vi "DrawTopMenuItems.vi"(7 "Collection in":refnum<class "Collection.lvclass">, 8 "error in (no error)":errorcluster, 10 "Coords":T2, 11 "Menu in":refnum<class "Menu.lvclass">) -> (0 "error out":errorcluster, 1 "SubMenu":bool, 2 "Area out":T1, 3 "Menu out":refnum<class "Menu.lvclass">, 4 "SelectedItemTeg":string, 5 "Collection out":refnum<class "Collection.lvclass">)   [LabVIEW 2021, in "Menu.lvlib" / "Menu.lvclass"]
uses:
  Menu.lvclass
  Menu.lvclass/Menu.ctl
  Picture2D/src/Text/Text.lvclass
  Picture2D/src/PointSpecialized/PointSpecialized.lvclass
  Picture2D/src/Rectangle/Rectangle.lvclass
  Picture2D/src/Collection/Collection.lvclass
  C:/GitHub/Picture2D/src/Point/Point.lvclass
  C:/GitHub/Picture2D/src/IDrawable/IDrawable.lvclass
  C:/GitHub/Picture2D/src/IMovable/IMovable.lvclass
  C:/GitHub/Picture2D/src/IRotatable/IRotatable.lvclass
  C:/GitHub/Picture2D/src/IScalable/IScalable.lvclass
  C:/GitHub/Picture2D/src/PointSpecialized/PointSpecialized.lvclass
  C:/GitHub/Picture2D/src/Polygone/Polygone.lvclass
  C:/GitHub/Picture2D/src/Shape/Shape.lvclass
  C:/GitHub/Picture2D/src/Picture2D/Picture2D.lvclass
  C:/GitHub/Picture2D/src/Rectangle/Rectangle.lvclass
  C:/GitHub/Picture2D/src/Text/Text.lvclass
  <vilib>/Utility/miscctls.llb/LVPoint32TypeDef.ctl
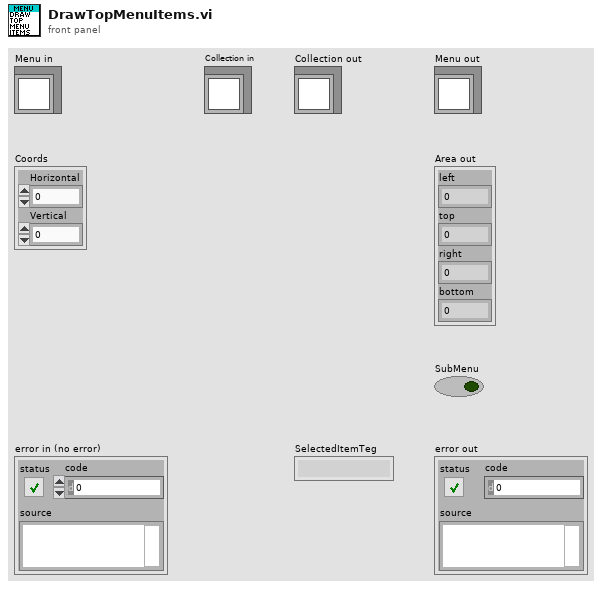
[diagram p1: front panel]
types:
  T1 = cluster{"left":i16, "top":i16, "right":i16, "bottom":i16}
  T2 = typedef "LVPoint32TypeDef.ctl" = cluster{"Horizontal":i32, "Vertical":i32}
  T3 = typedef "Menu.lvlib/Menu.lvclass/MenuItems.ctl" = cluster{"Item Name":string, "Short Cut":T4, "Checked":bool, "Enable":bool, "After item":string, "Item Tags":string[], "Item Names":string[], "Picture":refnum<class "Image.lvclass">, "Hilite Picture":refnum<class "Image.lvclass">, "Displayed":bool}
  T4 = typedef "LVMenuShortCut.ctl" = cluster{"Include Shift Key?":bool, "Include Ctrl Key?":bool, "Shortcut Key":string}
  T5 = typedef "Menu.lvlib/Menu.lvclass/MenuColors.ctl" = cluster{"Text":refnum<class "Color.lvclass">, "HiliteText":refnum<class "Color.lvclass">, "Background":refnum<class "Color.lvclass">, "BorderColor":refnum<class "Color.lvclass">, "Hilite":refnum<class "Color.lvclass">}
  T6 = enum16{"User-specified Font", "Application Font", "System Font", "Dialog Font"}
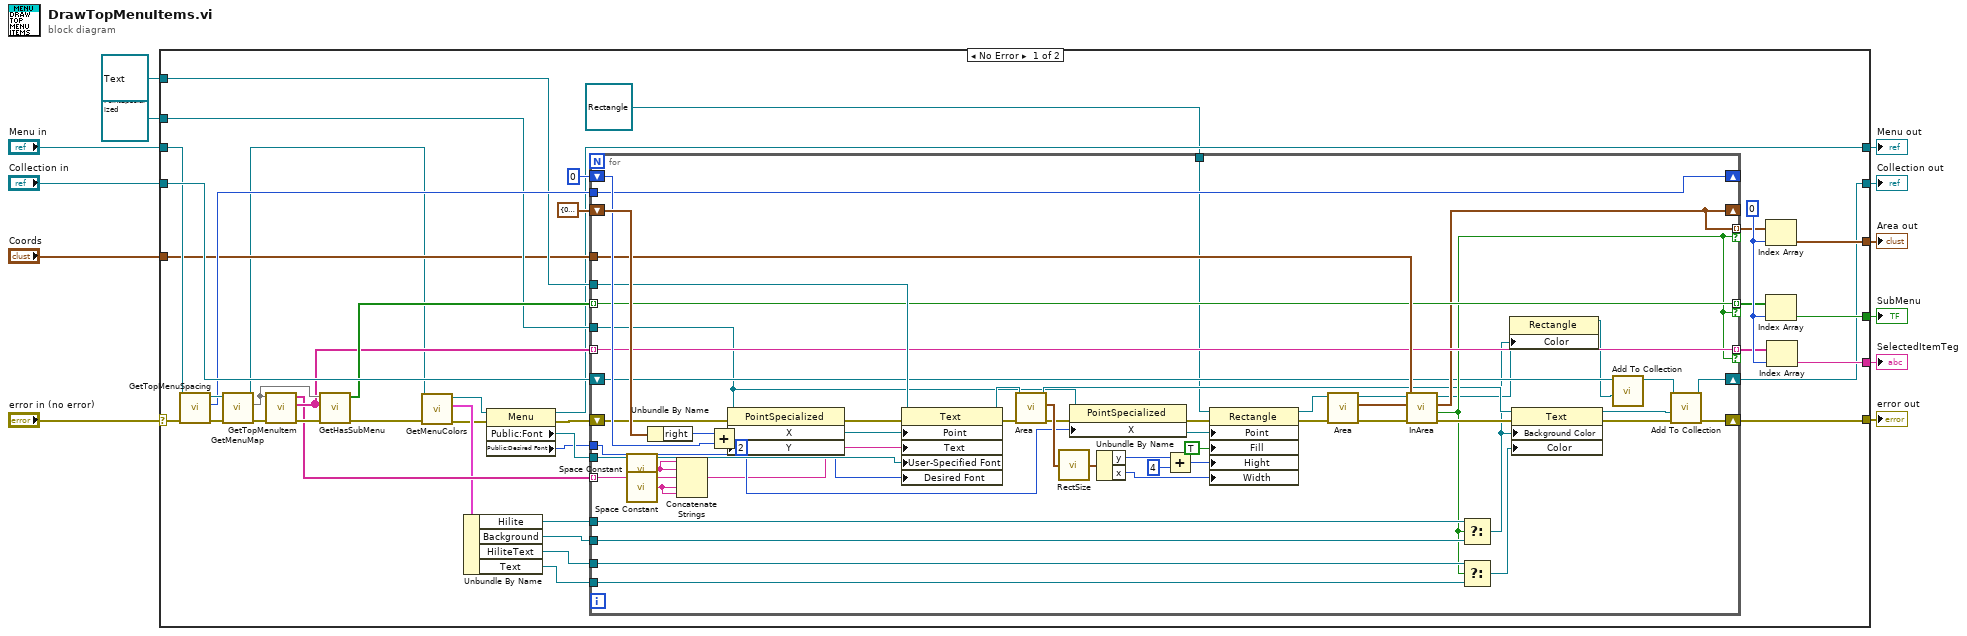
[diagram p0: block diagram]
diagram:
  n1 = case shown="No Error" "error in (no error)" {
    selector: "error in (no error)" -> [w43 w109]
    tunnel: [w16 w107] -> w11
    tunnel: "Collection in" -> [w52 w108]
    tunnel: [w49 w109] -> w9
    tunnel: "Menu in" -> [w44 w107]
    tunnel: [w42 _] -> w6
    tunnel: [w36 _] -> w5
    tunnel: [w34 _] -> w4
    tunnel: refnum<class "Text.lvclass"> refnum ("Picture2D.lvlib:Text") -> [w29 _]
    tunnel: "Coords" -> [w27 _]
    tunnel: [w28 w108] -> w1
    tunnel: refnum<class "PointSpecialized.lvclass"> refnum ("reference") -> [w30 _]
    frame No Error {
      w41 = 0 ("index")
      n2 = call "GetTopMenuSpacing.vi"("error in (no error)"=w43, "Menu in"=w44) -> ("error out"=w46:errorcluster, "TopMenuSpacing"=w45:i32, "Menu out"=w47:refnum<class "Menu.lvclass">)  [unwired: 7 in]
      n3 = call "GetMenuMap.vi"("error in (no error)"=w46, "Menu in"=w47) -> ("error out"=w50:errorcluster, "MenuMap"=w48:map{string, T3}, "Menu out"=w19:refnum<class "Menu.lvclass">)  [unwired: 7 in]
      n4 = call "GetTopMenuItem.vi"("error in (no error)"=w50, "MenuMap"=w48) -> ("error out"=w51:errorcluster, "Item Tags"=w38:string[], "Item Names"=w37:string[])  [unwired: 7 in]
      n5 = call "GetHasSubMenu.vi"("error in (no error)"=w51, "Item Tags"=w38, "MenuMap"=w48) -> ("error out"=w21:errorcluster, "HasSubMenu?"=w39:bool[])  [unwired: 7 in]
      n6 = call "GetMenuColors.vi"("error in (no error)"=w21, "Menu in"=w19) -> ("error out"=w20:errorcluster, "MenuColors"=w26:T5, "Menu out"=w17:refnum<class "Menu.lvclass">)  [unwired: 7 in]
      n7 = Unbundle By Name(w26) -> ("Hilite"=w22:refnum<class "Color.lvclass">, "Background"=w23:refnum<class "Color.lvclass">, "HiliteText"=w24:refnum<class "Color.lvclass">, "Text"=w25:refnum<class "Color.lvclass">)
      n8 = property class="Menu"(reference=w17, error in=w20) -> (reference out=w16:refnum<class "Menu.lvclass">, error out=w18:errorcluster, "Public:Font"=w15:refnum<class "Font.lvclass">, "Public:Desired Font"=w14:T6)
      n9 = for {
        tunnel: w37 -> [w80] mode=indexing
        shift-right: [w106] -> w28
        shift-left: w52 -> [w68]
        shift-right: [w85] -> _
        shift-left: T1 {"left"=0, "top"=0, "right"=0, "bottom"=0} ("Area out") -> [w104]
        tunnel: w23 -> [w100]
        tunnel: w22 -> [w97]
        tunnel: w25 -> [w99]
        tunnel: w24 -> [w98]
        tunnel: w27 -> [w95]
        tunnel: w29 -> [w94]
        tunnel: w30 -> [w57]
        shift-right: [w83] -> _
        shift-left: i16 0 ("Spacing") -> [w102]
        tunnel: w45 -> [w83]
        tunnel: [w93] -> w33 mode=indexing if=w84
        tunnel: [w85] -> w35 mode=indexing if=w84
        tunnel: w38 -> [w93] mode=indexing
        tunnel: w39 -> [w92] mode=indexing
        tunnel: [w92] -> w40 mode=indexing if=w84
        shift-right: [w88] -> w49
        shift-left: w18 -> [w91]
        tunnel: w15 -> [w82]
        tunnel: w14 -> [w81]
        tunnel: refnum<class "Rectangle.lvclass"> refnum ("reference") -> [w65]
        n10 = call <vilib>:"Space Constant.vi"() -> ("String"=w53:string)
        n11 = call <vilib>:"Space Constant.vi"() -> ("String"=w54:string)
        n12 = Unbundle By Name(w104) -> ("right"=w103:i16)
        n13 = Concatenate Strings(w53, w53, w80, w54, w54) -> (w58:string)
        n14 = Add(x=w103, y=w102) -> (x+y=w59:i32)
        n15 = property class="PointSpecialized"(reference=w57, error in=w91, "X"=w59, "Y"=i16 2 ("Point:y")) -> (reference out=w56:refnum<class "PointSpecialized.lvclass">, error out=w90:errorcluster)
        n16 = property class="Text"(reference=w94, error in=w90, "Point"=w56, "Text"=w58, "User-Specified Font"=w82, "Desired Font"=w81) -> (reference out=w72:refnum<class "Text.lvclass">, error out=w71:errorcluster)
        n17 = call-dynamic "Area.vi"("error in (no error)"=w71, "Text in"=w72) -> ("error out"=w74:errorcluster, "rect"=w77:T1, "Text out"=w66:refnum<class "Text.lvclass">)  [unwired: 7 in]
        n18 = call <vilib>:"RectSize.vi"("rect"=w77) -> ("point"=w78:cluster{"x":i16, "y":i16})
        n19 = property class="PointSpecialized"(reference=w57, "X"=w59) -> (reference out=w55:refnum<class "PointSpecialized.lvclass">)  [unwired: 1 in, 1 out]
        n20 = Unbundle By Name(w78) -> ("y"=w61:i16, "x"=w69:i16)
        n21 = Add(x=w61, y=i16 4) -> (x+y=w76:i16)
        n22 = property class="Rectangle"(reference=w65, error in=w74, "Point"=w55, "Fill"=TRUE, "Hight"=w76, "Width"=w69) -> (reference out=w73:refnum<class "Rectangle.lvclass">, error out=w70:errorcluster)
        n23 = call-dynamic "Area.vi"("error in (no error)"=w70, "Rectangle in"=w73) -> ("error out"=w87:errorcluster, "rect"=w105:T1, "Rectangle out"=w64:refnum<class "Rectangle.lvclass">)  [unwired: 7 in]
        n24 = call "InArea.vi"("error in (no error)"=w87, "Area in"=w105, "Coords"=w95) -> ("error out"=w86:errorcluster, "InArea"=w84:bool, "Area out"=w85:T1)  [unwired: 6 in]
        n25 = Select(t=w97, s=w84, f=w100) -> (s? t:f=w62:refnum<class "Color.lvclass">)
        n26 = Select(t=w98, s=w84, f=w99) -> (s? t:f=w96:refnum<class "Color.lvclass">)
        n27 = property class="Rectangle"(reference=w64, "Color"=w62) -> (reference out=w63:refnum<class "Rectangle.lvclass">)  [unwired: 1 in, 1 out]
        n28 = property class="Text"(reference=w66, error in=w86, "Background Color"=w62, "Color"=w96) -> (reference out=w101:refnum<class "Text.lvclass">, error out=w89:errorcluster)
        n29 = call-dynamic "Add To Collection.vi"("IDrawable"=w63, "Collection in"=w68) -> ("Collection out"=w67:refnum<class "Collection.lvclass">)  [unwired: 8 in, 1 out]
        n30 = call-dynamic "Add To Collection.vi"("error in (no error)"=w89, "IDrawable"=w101, "Collection in"=w67) -> ("error out"=w88:errorcluster, "Collection out"=w106:refnum<class "Collection.lvclass">)  [unwired: 7 in]
      }
      n31 = Index Array(array=w35, index=w41) -> (element=w36:T1)
      n32 = Index Array(array=w40, index=w41) -> (element=w42:bool)
      n33 = Index Array(array=w33, index=w41) -> (element=w34:string)
    }
    frame Error {
    }
  }
  "Menu out" <- w11
  "error out" <- w9
  "SubMenu" <- w6
  "Area out" <- w5
  "SelectedItemTeg" <- w4
  "Collection out" <- w1
